vi "Reboot Test.vi"() -> ()   [LabVIEW 2019]
uses:
  PF_API.lvclass
panel:
  in  "Parameter Value":string[](array[string])
  in  "Parameter Key":string[](array[string])
  in  "Command String":string="get_parameter"
  out "body":string
  in  "Scanner IP Address":string
  in  "Host IP Address":string
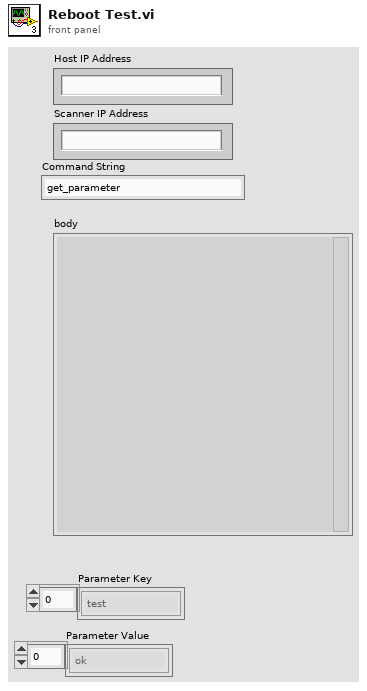
[diagram p1: front panel]
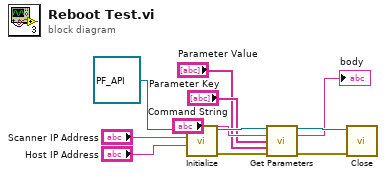
[diagram p0: block diagram]
diagram:
  n1 = call-dynamic "Initialize.vi"("Host IP Address"="Host IP Address", "Scanner IP Address"="Scanner IP Address", "PF_API in"=refnum<class "PF_API.lvclass"> refnum) -> ("error out"=w11:errorcluster, "PF_API out"=w6:refnum<class "PF_API.lvclass">)  [unwired: 7 in]
  n2 = call-dynamic "Get Parameters.vi"("PF_API in"=w6, "Command String"="Command String", "Parameter Key"="Parameter Key", "Parameter Value"="Parameter Value", "error in (no error)"=w11) -> ("PF_API out"=w5:refnum<class "PF_API.lvclass">, "body"=→"body":string, "error out"=w7:errorcluster)  [unwired: 8 in]
  n3 = call-dynamic "Close.vi"("error in (no error)"=w7, "PF_API in"=w5) -> ()  [unwired: 8 in, 2 out]
